vi "四人表决电路设计.vi"() -> ()   [LabVIEW 2018]
panel:
  in  "结束":bool
  out "布尔":bool
  in  "D":bool
  in  "C":bool
  in  "B":bool
  in  "A":bool
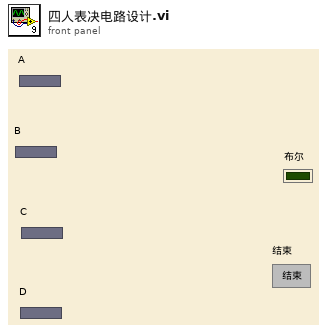
[diagram p1: front panel]
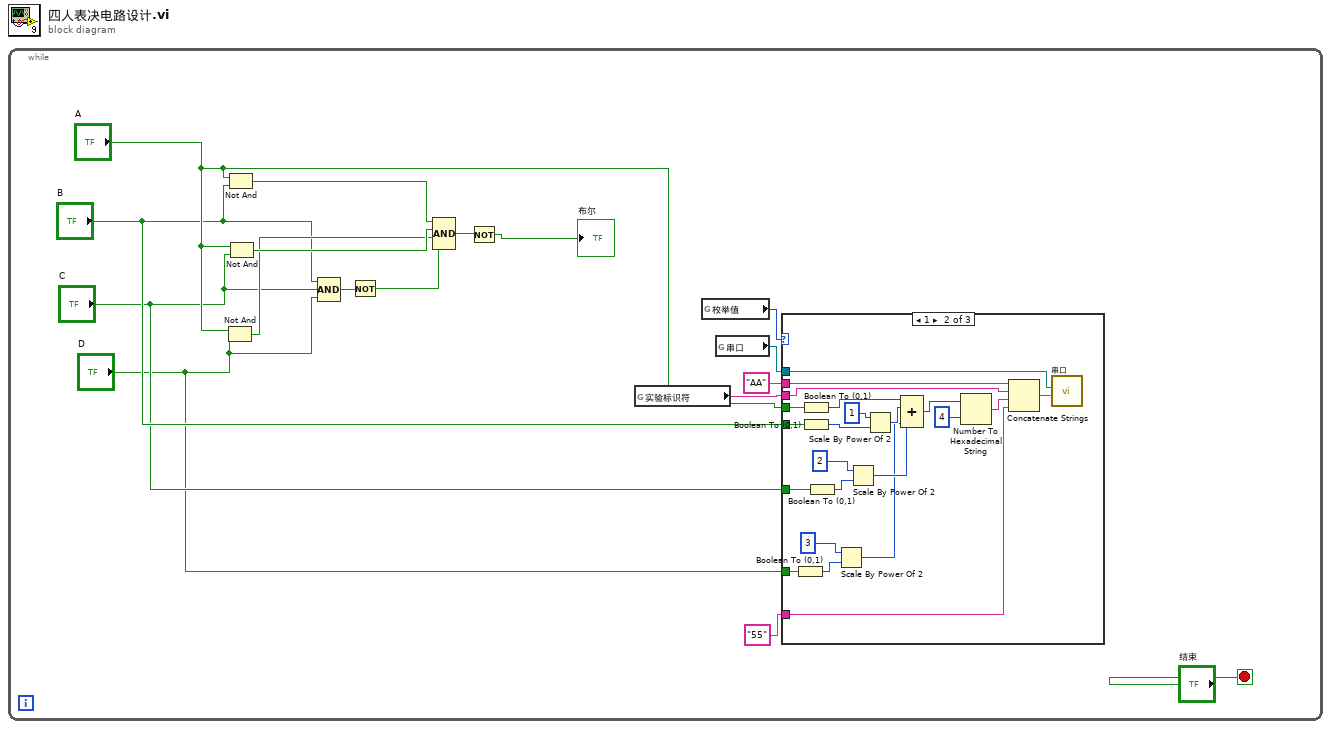
[diagram p0: block diagram]
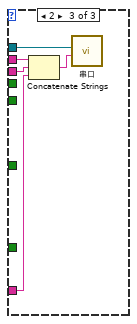
[diagram p3: hidden frame]
diagram:
  n1 = while {
    stop <- "结束" stop-if-true
    n2 = Not And(1:"D", 2:"A") -> (0:w13:bool)
    n3 = Not And(1:"B", 2:"A") -> (0:w15:bool)
    n4 = Not And(1:"C", 2:"A") -> (0:w14:bool)
    n5 = Compound Arithmetic op=AND ("复合运算")("B", "C", "D") -> (w17:bool)
    n6 = Not(x=w17) -> (.not. x?=w12:bool)
    n7 = Compound Arithmetic op=AND ("复合运算")(w15, w14, w13, w12) -> (w16:bool)
    n8 = Not(x=w16) -> (.not. x?=→"布尔":bool)
    n9 = global read "全局变量.vi" "实验标识符"() -> (w7:string)
    n10 = global read "全局变量.vi" "枚举值"() -> (w9:i8)
    n11 = global read "全局变量.vi" "串口"() -> (w8:refnum<visa-resource-name>)
    n12 = case shown="1" w9 {
      tunnel: "B" -> [_ w34 _]
      tunnel: "A" -> [_ w33 _]
      tunnel: w8 -> [_ w32 w42]
      tunnel: w7 -> [_ w31 w43]
      tunnel: "55" -> [_ w30 w40]
      tunnel: "AA" -> [_ w29 w41]
      tunnel: "C" -> [_ w23 _]
      tunnel: "D" -> [_ w18 _]
      frame 0, Default {
      }
      frame 1 {
        n13 = Boolean To (0,1)(Boolean=w18) -> (0, 1=w21:i16)
        n14 = Boolean To (0,1)(Boolean=w33) -> (0, 1=w38:i16)
        n15 = Boolean To (0,1)(Boolean=w34) -> (0, 1=w36:i16)
        n16 = Boolean To (0,1)(Boolean=w23) -> (0, 1=w24:i16)
        n17 = Scale By Power Of 2(n=3, x=w21) -> (x*2^n=w19:i16)
        n18 = Scale By Power Of 2(n=2, x=w24) -> (x*2^n=w25:i16)
        n19 = Scale By Power Of 2(n=1, x=w36) -> (x*2^n=w37:i16)
        n20 = Compound Arithmetic op=ADD ("复合运算")(w38, w37, w25, w19) -> (w28:i16)
        n21 = Number To Hexadecimal String(1:4, 2:w28) -> (0:w26:string)
        n22 = Concatenate Strings(w29, w31, w26, w30) -> (w39:string)
        n23 = call "串口.vi"("字符串"=w39, "VISA resource name"=w32) -> ()  [unwired: 10 in]
      }
      frame 2 {
        n24 = Concatenate Strings(w41, w43, w40) -> (w44:string)
        n25 = call "串口.vi"("字符串"=w44, "VISA resource name"=w42) -> ()  [unwired: 10 in]
      }
    }
  }
